vi "GVISA Mux Open.vi"(8 "error in":errorcluster, 11 "session in":T1={"VISA"="", "paths"=[], "idn command"="", "serial cfg"={"Baud rate"=9600, "Data bits"=8, "Parity"=0, "Stop bits"=10, "Flow control"=0, "End Mode Read"=enum."None", "End Mode Write"=enum."None", "Term character"=0, "Term enable"=FALSE}} {"serial cfg"."Flow control" items=["None", "XON/XOFF", "CTS/RTS", "XON/XOFF + CTS/RTS", "DTR/DSR", "XON/XOFF + DTR/DSR"]; "serial cfg"."Stop bits" items=["1 bit"=10, "1.5 bits"=15, "2 bits"=20]; "serial cfg"."Parity" items=["None", "Odd", "Even", "Mark", "Space"]; "serial cfg"."Data bits" items=["5 bits"=5, "6 bits"=6, "7 bits"=7, "8 bits"=8]; "serial cfg"."Baud rate" items=["150 Bd"=150, "300 Bd"=300, "600 Bd"=600, "1200 Bd"=1200, "2400 Bd"=2400, "4800 Bd"=4800, "9600 Bd"=9600, "19.2 kBd"=19200, "38.4 kBd"=38400, "57.6 kBd"=57600, "115.2 kBd"=115200]}) -> (0 "error out":errorcluster, 2 "idn string":string, 3 "session out":T1={"VISA"="", "paths"=[], "idn command"="", "serial cfg"={"Baud rate"=9600, "Data bits"=8, "Parity"=0, "Stop bits"=10, "Flow control"=0, "End Mode Read"=enum."None", "End Mode Write"=enum."None", "Term character"=0, "Term enable"=FALSE}} {"serial cfg"."Flow control" items=["None", "XON/XOFF", "CTS/RTS", "XON/XOFF + CTS/RTS", "DTR/DSR", "XON/XOFF + DTR/DSR"]; "serial cfg"."Stop bits" items=["1 bit"=10, "1.5 bits"=15, "2 bits"=20]; "serial cfg"."Parity" items=["None", "Odd", "Even", "Mark", "Space"]; "serial cfg"."Data bits" items=["5 bits"=5, "6 bits"=6, "7 bits"=7, "8 bits"=8]; "serial cfg"."Baud rate" items=["150 Bd"=150, "300 Bd"=300, "600 Bd"=600, "1200 Bd"=1200, "2400 Bd"=2400, "4800 Bd"=4800, "9600 Bd"=9600, "19.2 kBd"=19200, "38.4 kBd"=38400, "57.6 kBd"=57600, "115.2 kBd"=115200]})   [LabVIEW 2020]
doc: "Opens generic VISA command mutiplexer. If IDN command is not empty, it will try to send and read answer as idn string. Otherwise it will return default 'Generic VISA multiplexer'. It also sets COM port baud and stuff if serial VISA."
uses:
  GVISA Mux Session.ctl
  GVISA Mux Path Entry.ctl
  met_serial_setup.ctl
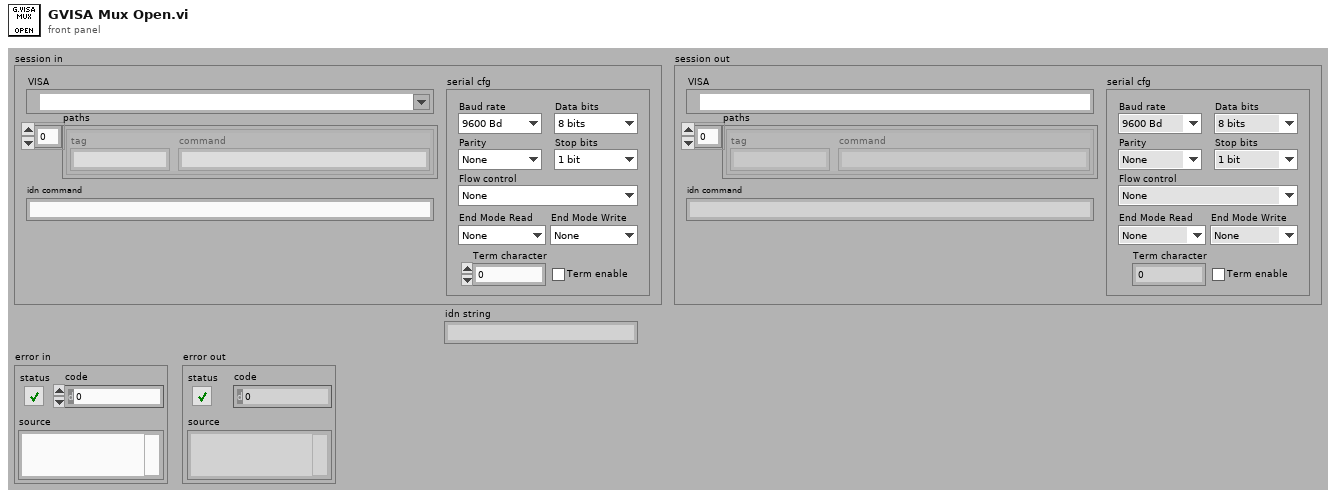
[diagram p1: front panel]
types:
  T1 = typedef "GVISA Mux Session.ctl" = cluster{"VISA":refnum<visa-resource-name>, "paths":T2[], "idn command":string, "serial cfg":T3}
  T2 = typedef "GVISA Mux Path Entry.ctl" = cluster{"tag":string, "command":string}
  T3 = typedef "met_serial_setup.ctl" = cluster{"Baud rate":i32, "Data bits":i32, "Parity":i32, "Stop bits":i32, "Flow control":i32, "End Mode Read":enum16{"None", "Last Bit", "TermChar"}, "End Mode Write":enum16{"None", "Last Bit", "TermChar"}, "Term character":u8, "Term enable":bool}
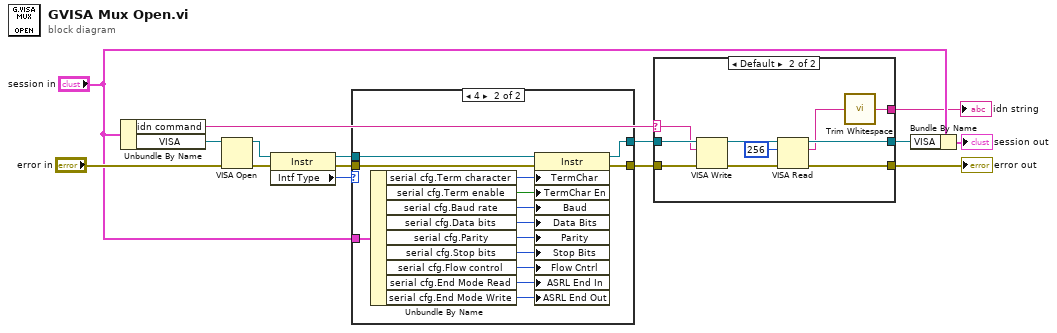
[diagram p0: block diagram]
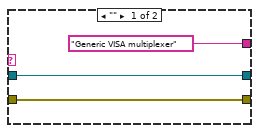
[diagram p3: hidden frame]
diagram:
  n1 = Unbundle By Name("session in") -> ("idn command"=w13:string, "VISA"=w14:refnum<visa-resource-name>)
  n2 = VISA Open(error in (no error)="error in", VISA resource name=w14) -> (VISA resource name=w10:refnum<visa-resource-name>, error out=w11:errorcluster)  [unwired: 3 in]
  n3 = property class="Instr"(reference=w10, error in=w11) -> (reference out=w7:refnum<visa-resource-name>, error out=w8:errorcluster, "Intf Type"=w9:u16)
  n4 = case shown="4" w9 {
    tunnel: w8 -> [w17 w31]
    tunnel: w7 -> [w16 w30]
    tunnel: "session in" -> [_ w29]
    tunnel: [w17 w19] -> w6
    tunnel: [w16 w18] -> w5
    frame 0, Default {
    }
    frame 4 {
      n5 = Unbundle By Name(w29) -> ("serial cfg.Term character"=w21:u8, "serial cfg.Term enable"=w20:bool, "serial cfg.Baud rate"=w28:i32, "serial cfg.Data bits"=w27:i32, "serial cfg.Parity"=w26:i32, "serial cfg.Stop bits"=w25:i32, "serial cfg.Flow control"=w24:i32, "serial cfg.End Mode Read"=w23:enum16{"None", "Last Bit", "TermChar"}, "serial cfg.End Mode Write"=w22:enum16{"None", "Last Bit", "TermChar"})
      n6 = property class="Instr"(reference=w30, error in=w31, "TermChar"=w21, "TermChar En"=w20, "Baud"=w28, "Data Bits"=w27, "Parity"=w26, "Stop Bits"=w25, "Flow Cntrl"=w24, "ASRL End In"=w23, "ASRL End Out"=w22) -> (reference out=w18:refnum<visa-resource-name>, error out=w19:errorcluster)
    }
  }
  n7 = case shown="Default" w13 {
    selector: w13 -> [_ w42]
    tunnel: w6 -> [w33 w44]
    tunnel: w5 -> [w34 w43]
    tunnel: [w33 w38] -> w12
    tunnel: [w34 w37] -> w3
    tunnel: ["Generic VISA multiplexer" ("trimmed string") w35] -> w1
    frame "" {
    }
    frame Default {
      n8 = VISA Write(VISA resource name=w43, write buffer=w42, error in (no error)=w44) -> (VISA resource name out=w40:refnum<visa-resource-name>, error out=w41:errorcluster)  [unwired: 1 out]
      n9 = VISA Read(VISA resource name=w40, byte count=u32 256, error in (no error)=w41) -> (VISA resource name out=w37:refnum<visa-resource-name>, read buffer=w36:string, error out=w38:errorcluster)  [unwired: 1 out]
      n10 = call <vilib>:"Trim Whitespace.vi"("string"=w36) -> ("trimmed string"=w35:string)  [unwired: 1 in]
    }
  }
  "error out" <- w12
  "idn string" <- w1
  n11 = Bundle By Name(cluster="session in", "VISA"=w3) -> (→"session out":T1)
